vi "Extract Palette Information.vi"() -> ()   [LabVIEW 2019]
doc: "Illustrates how to read data from an existing .mnu file."
uses:
  <vilib>/Palette API/Palette Menu/Public Type Define/Palette type.ctl
  <vilib>/Palette API/Palette Menu/Palette Menu.lvlib
panel:
  out "Palette Display Name":string
  out "Palette Icon":picture
  # "Overview: Demonstrates the use of the Palette Editing VIs to read information about an existing palette.\nInstructions:\n1. Make sure you have already run the Create New Palette.vi example.\n2. Run this VI. It will display the name and icon of the PaletteAPI.mnu palette."
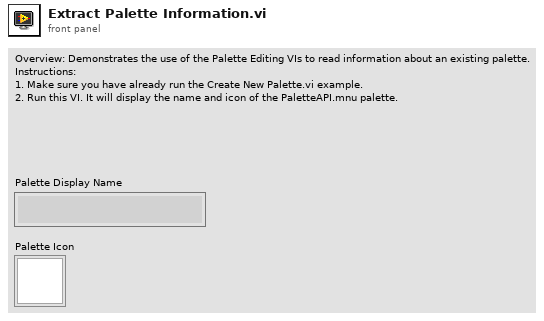
[diagram p1: front panel]
types:
  T1 = typedef "Palette Menu.lvlib/Palette type.ctl" = i32
  T2 = typedef "Palette Menu.lvlib/Palette Data.ctl" = cluster{"display name":string, "view format":T3, "palette width":i16, "items":T4, "256 color icon":picture, "B&W color icon":picture, "help information":T6, "palette description":string, "synchronize information":T7}
  T3 = typedef "Palette Menu.lvlib/View Format.ctl" = u16
  T4 = typedef "Palette Menu.lvlib/Items.ctl" = T5[]
  T5 = typedef "Palette Menu.lvlib/Item.ctl" = cluster{"item path":path, "library path":path, "use default lvlib palette":bool, "short name":string, "place VI contents":bool, "hide synchronized item":bool, "reserve spot for synch item":bool, "configure when placing VI contents":bool}
  T6 = typedef "Palette Menu.lvlib/Help Info.ctl" = cluster{"help tag":string, "help file path ":path}
  T7 = typedef "Palette Menu.lvlib/Synchronize Info.ctl" = cluster{"synchronize with directory":bool, "synchronize directory path":path}
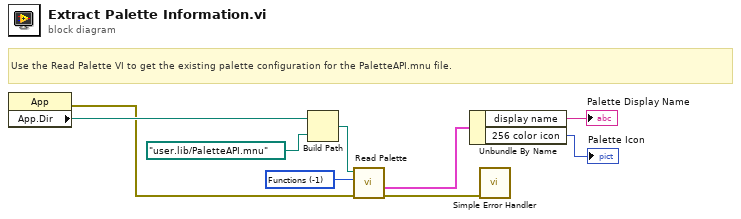
[diagram p0: block diagram]
diagram:
  w5 = T1 -1 items=["Functions"=-1, "Controls"=-2] ("palette type")
  # "Use the Read Palette VI to get the existing palette configuration for the PaletteAPI.mnu file."
  n1 = property class="App"() -> (error out=w1:errorcluster, "App.Dir"=w3:path)  [unwired: 2 in, 1 out]
  n2 = Build Path(base path=w3, name or relative path=path "user.lib/PaletteAPI.mnu") -> (appended path=w4:path)
  n3 = call <vilib>:"Read Palette.vi"("error in (no error)"=w1, "palette type"=w5, "palette path"=w4) -> ("error out"=w9:errorcluster, "palette data"=w8:T2)  [unwired: 1 in, 6 out]
  n4 = Unbundle By Name(w8) -> ("display name"=→"Palette Display Name":string, "256 color icon"=→"Palette Icon":picture)
  n5 = call <vilib>:"Simple Error Handler.vi"("error in (no error)"=w9) -> ()  [unwired: 1 in, 8 out]
